vi "stackErrorSimpleMulti.vi"(1 "Error List":u32[](array[numeric])) -> (0 "Error Out":u32)   [LabVIEW 2021]
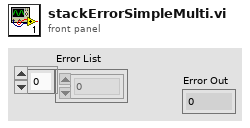
[diagram p1: front panel]
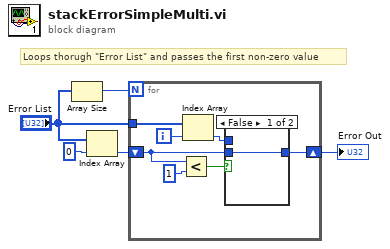
[diagram p0: block diagram]
diagram:
  # "Loops thorugh \"Error List\" and passes the first non-zero value"
  n1 = Array Size(array="Error List") -> (size(s)=w5:i32)
  n2 = Index Array(array="Error List", index=0) -> (element=w3:u32)
  n3 = for {
    N: w5 -> [_]
    tunnel: "Error List" -> [w11]
    shift-right: [w6] -> w2
    shift-left: w3 -> [w7]
    i -> [w12]
    n4 = Less?(x=w7, y=1) -> (x < y?=w9:bool)
    n5 = Index Array(array=w11, index=w12) -> (element=w8:u32)
    n6 = case shown="False" w9 {
      tunnel: w8 -> [_ w14]
      tunnel: [w13 w14] -> w6
      tunnel: w7 -> [w13 _]
      frame False {
      }
      frame True {
      }
    }
  }
  "Error Out" <- w2
